vi "Append unique suffix -- V1.vi"(6 "Extention":string, 7 "Suffix":string, 8 "error in (no error)":errorcluster, 10 "ovewrite ?":bool, 11 "Path":path) -> (0 "error out":errorcluster, 3 "Path out":path)   [LabVIEW 2021]
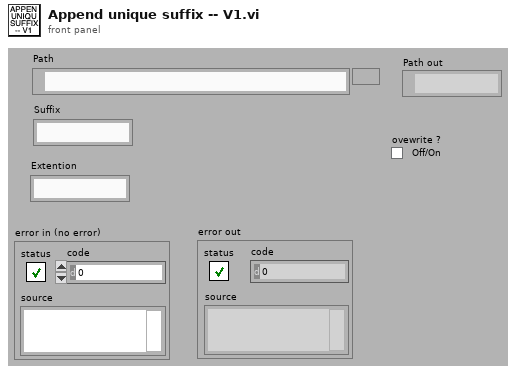
[diagram p1: front panel]
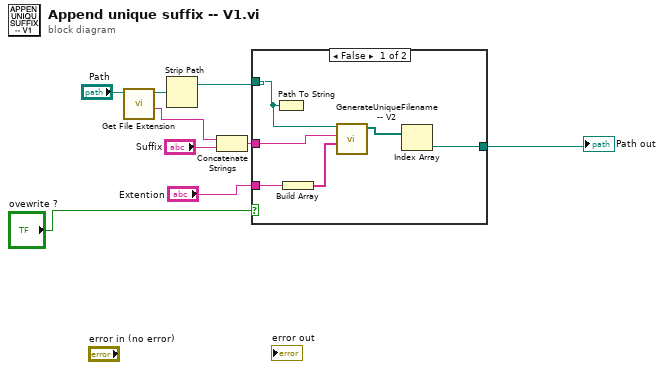
[diagram p0: block diagram]
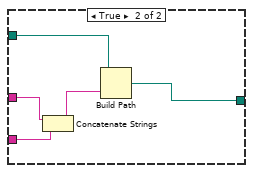
[diagram p2: hidden frame]
diagram:
  n1 = call <vilib>:"Get File Extension.vi"("file"="Path") -> ("filename without extension"=w4:string, "dup file"=w3:path)  [unwired: 6 in, 3 out]
  n2 = Strip Path(path=w3) -> (stripped path=w6:path)  [unwired: 1 out]
  n3 = Concatenate Strings(w4, "Suffix") -> (w8:string)
  n4 = case shown="False" "ovewrite ?" {
    tunnel: w8 -> [w15 w20]
    tunnel: "Extention" -> [w14 w19]
    tunnel: w6 -> [w10 w18]
    tunnel: [w11 w16] -> w2
    frame False {
      n5 = Path To String(path=w10) -> ()  [unwired: 1 out]
      n6 = Build Array(w14) -> (w13:string[])
      n7 = call "GenerateUniqueFilename -- V2.vi"("File Name Suffixes"=w13, "File Name Prefix"=w15, "Folder"=w10) -> ("Paths"=w12:path[])  [unwired: 7 in, 1 out]
      n8 = Index Array(array=w12) -> (element=w11:path)  [unwired: 1 in]
    }
    frame True {
      n9 = Concatenate Strings(w20, w19) -> (w17:string)
      n10 = Build Path(base path=w18, name or relative path=w17) -> (appended path=w16:path)
    }
  }
  "Path out" <- w2
